vi "DJGuetta (3).vi"() -> ()   [LabVIEW 2018]
uses:
  EdoDJGuetta.ctl
panel:
  out "PteVer":i32
  out "PteHor":i32
  out "String":string
  in  "Start":bool
  out "PVer":i32
  out "PHor":i32
  in  "stop":bool
  in  "BHor":bool
  in  "BVer":bool
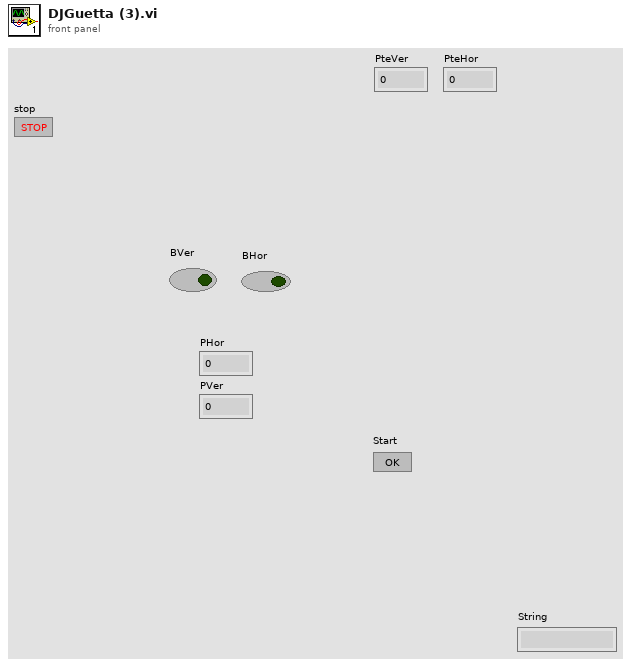
[diagram p1: front panel]
types:
  T1 = typedef "EdoDJGuetta.ctl" = enum16{"Inicio", "Baja1", "Pausa1", "Sube1", "Pausa2", "Derecha", "Pausa3", "Baja2", "Pausa4", "Sube2", "Pausa5", "Izq", "Pausa6", "Fin"}
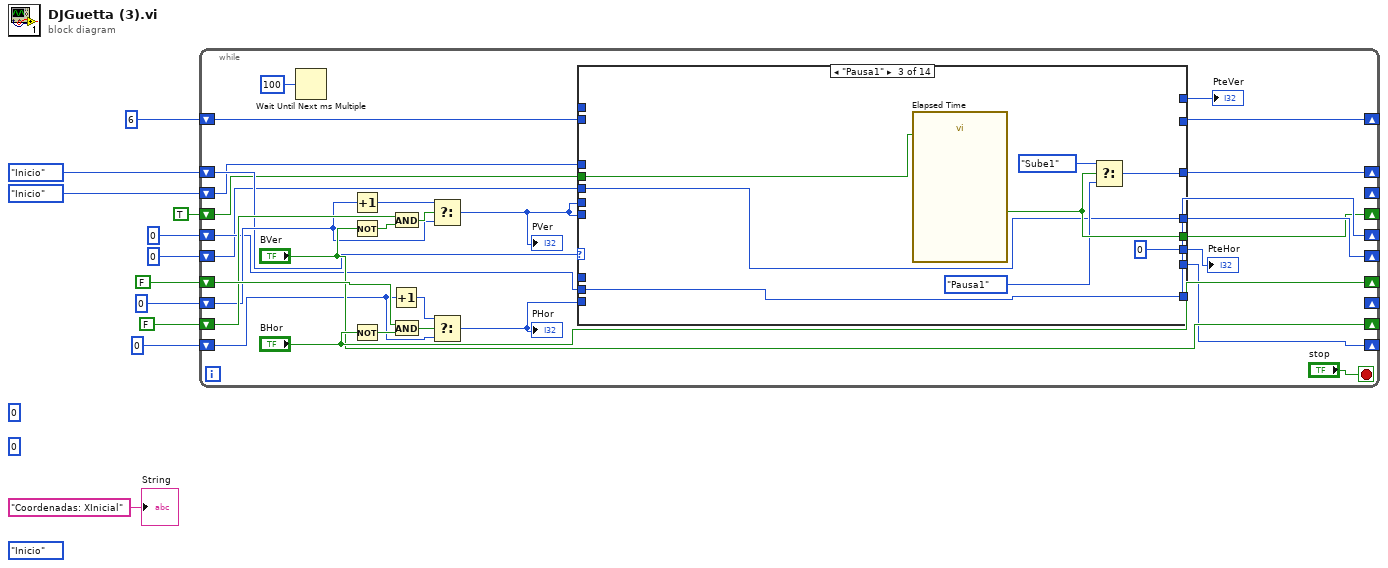
[diagram p0: block diagram]
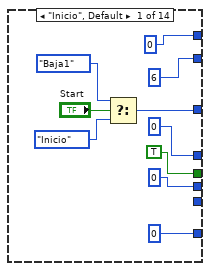
[diagram p2: hidden frame]
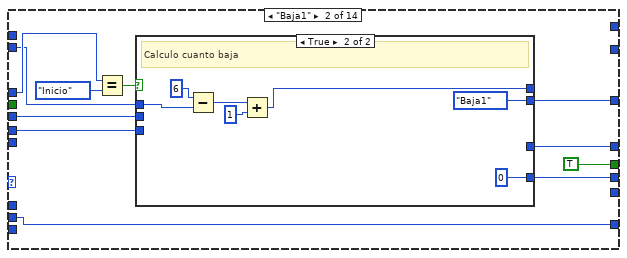
[diagram p3: hidden frame]
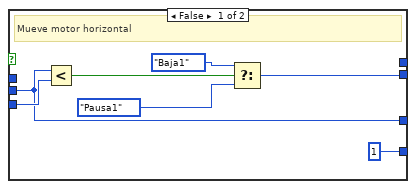
[diagram p4: hidden frame]
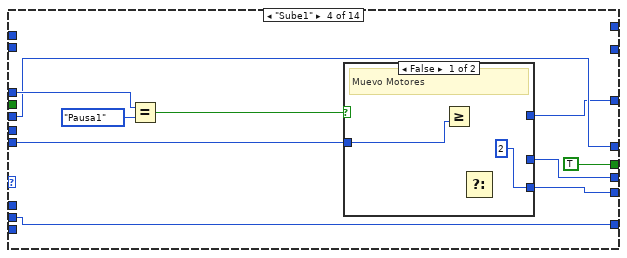
[diagram p5: hidden frame]
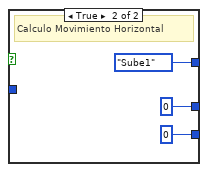
[diagram p6: hidden frame]
diagram:
  (unwired) EdoDJGuetta."Inicio"
  (unwired) 0
  (unwired) 0
  n1 = while {
    shift-right: ["BHor"] -> _
    shift-left: FALSE -> [w37]
    shift-right: ["BVer"] -> _
    shift-left: FALSE -> [w34]
    shift-right: [w16] -> _
    shift-left: 0 -> [w31]
    shift-right: _ -> [_]
    shift-left: 0 -> [w28]
    shift-right: [w21] -> _
    shift-left: EdoDJGuetta."Inicio" -> [w27]
    shift-right: [w13] -> _
    shift-left: 6 -> [w26]
    shift-right: [w24] -> _
    shift-left: 0 -> [w25]
    shift-right: [w22] -> _
    shift-left: 0 -> [w23]
    shift-right: _ -> [_]
    shift-left: EdoDJGuetta."Inicio" -> [w20]
    shift-right: [w17] -> _
    shift-left: TRUE -> [w18]
    stop <- "stop" stop-if-true
    n2 = Wait Until Next ms Multiple(millisecond multiple=u32 100) -> ()  [unwired: 1 out]
    n3 = Increment(x=w28) -> (x+1=w29:i32)
    n4 = Not(x="BVer") -> (.not. x?=w38:bool)
    n5 = Not(x="BHor") -> (.not. x?=w39:bool)
    n6 = Increment(x=w31) -> (x+1=w32:i32)
    n7 = And(x=w34, y=w38) -> (x .and. y?=w30:bool)
    n8 = And(x=w37, y=w39) -> (x .and. y?=w33:bool)
    n9 = Select(t=w29, s=w30, f=w28) -> (s? t:f=w14:i32)
    "PVer" <- w14
    n10 = Select(t=w32, s=w33, f=w31) -> (s? t:f=w15:i32)
    "PHor" <- w15
    n11 = case shown="\"Pausa1\"" w27 {
      tunnel: _ -> [_ _ w79 w94 _ _ _ _ _ _ _ _ _ _]
      tunnel: w26 -> [_ w58 w78 w93 _ _ _ _ _ _ _ _ _ _]
      tunnel: w25 -> [_ w59 w80 w92 _ _ _ _ _ _ _ _ _ _]
      tunnel: [0 w59 w80 w92 _ _ _ _ _ _ _ _ _ _] -> w24
      tunnel: _ -> [_ _ w82 w91 _ _ _ _ _ _ _ _ _ _]
      tunnel: w23 -> [_ w56 w81 w96 _ _ _ _ _ _ _ _ _ _]
      tunnel: [0 w55 w81 w96 _ _ _ _ _ _ _ _ _ _] -> w22
      tunnel: [w49 w57 w83 w95 _ _ _ _ _ _ _ _ _ _] -> w21
      tunnel: w20 -> [_ w62 _ w97 _ _ _ _ _ _ _ _ _ _]
      tunnel: w14 -> [_ w54 _ _ _ _ _ _ _ _ _ _ _ _]
      tunnel: [0 w53 0 w89 _ _ _ _ _ _ _ _ _ _] -> w19
      tunnel: w18 -> [_ _ w87 _ _ _ _ _ _ _ _ _ _ _]
      tunnel: [TRUE ("Time has Elapsed") TRUE ("Time has Elapsed") w86 TRUE ("Time has Elapsed") _ _ _ _ _ _ _ _ _ _] -> w17
      tunnel: [_ _ _ w98 _ _ _ _ _ _ _ _ _ _] -> w16
      tunnel: w15 -> [_ _ _ _ _ _ _ _ _ _ _ _ _ _]
      tunnel: w14 -> [_ _ _ w88 _ _ _ _ _ _ _ _ _ _]
      tunnel: [6 _ _ _ _ _ _ _ _ _ _ _ _ _] -> w13
      tunnel: [0 _ _ _ _ _ _ _ _ _ _ _ _ _] -> w12
      frame "Inicio", Default {
        n12 = Select(t=EdoDJGuetta."Baja1", s="Start", f=EdoDJGuetta."Inicio") -> (s? t:f=w49:T1)
      }
      frame "Baja1" {
        n13 = Equal?(x=w62, y=EdoDJGuetta."Inicio") -> (x = y?=w60:bool)
        n14 = case shown="True" w60 {
          tunnel: w58 -> [_ w75]
          tunnel: [_ w72] -> _
          tunnel: [w66 EdoDJGuetta."Baja1"] -> w57
          tunnel: w56 -> [w63 _]
          tunnel: [w63 _] -> w55
          tunnel: w54 -> [w65 _]
          tunnel: [1 0] -> w53
          frame False {
            # "Mueve motor horizontal"
            n15 = Less?(x=w63, y=w65) -> (x < y?=w68:bool)
            n16 = Select(t=EdoDJGuetta."Baja1", s=w68, f=EdoDJGuetta."Pausa1") -> (s? t:f=w66:T1)
          }
          frame True {
            # "Calculo cuanto baja"
            n17 = Subtract(x=6, y=w75) -> (x-y=w74:i32)
            n18 = Add(x=w74, y=1) -> (x+y=w72:i32)
          }
        }
      }
      frame "Pausa1" {
        n19 = call "Elapsed Time"("Reset"=w87) -> ("Time has Elapsed"=w86:bool)  [unwired: 11 in, 7 out]
        n20 = Select(t=EdoDJGuetta."Sube1", s=w86, f=EdoDJGuetta."Pausa1") -> (s? t:f=w83:T1)
      }
      frame "Sube1" {
        n21 = Equal?(x=w97, y=EdoDJGuetta."Pausa1") -> (x = y?=w99:bool)
        n22 = case shown="False" w99 {
          tunnel: [2 0] -> w98
          tunnel: [_ EdoDJGuetta."Sube1"] -> w95
          tunnel: [_ 0] -> w89
          tunnel: w88 -> [w102 _]
          frame False {
            # "Muevo Motores"
            n23 = Greater Or Equal?(y=w102) -> ()  [unwired: 1 in, 1 out]
            n24 = Select() -> ()  [unwired: 3 in, 1 out]
          }
          frame True {
            # "Calculo Movimiento Horizontal"
          }
        }
      }
      frame "Pausa2" {
      }
      frame "Derecha" {
      }
      frame "Pausa3" {
      }
      frame "Baja2" {
      }
      frame "Pausa4" {
      }
      frame "Sube2" {
      }
      frame "Pausa5" {
      }
      frame "Izq" {
      }
      frame "Pausa6" {
      }
      frame "Fin" {
      }
    }
    "PteHor" <- w19
    "PteVer" <- w12
  }
  "String" <- "Coordenadas: XInicial"
